vi "Set Enable Generic Event Flag.vi"(10 "Enable Generic Event Flag":bool, 11 "Template Server in":refnum<class "Template Server.lvclass">) -> (3 "Template Server out":refnum<class "Template Server.lvclass">)   [LabVIEW 2019, in "Template Server.lvlib" / "Template Server.lvclass"]
doc: "Enable the generic event if you would like to use a single event for capturing all messages. This would be useful if you are planning to implement your own dispatcher logic.\n\nKindly note that if generic event is enabled, individual events won't get generated."
uses:
  Template Server.lvclass
  Template Server.lvclass/Template Server.ctl
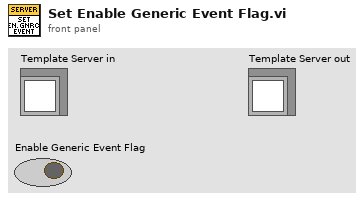
[diagram p1: front panel]
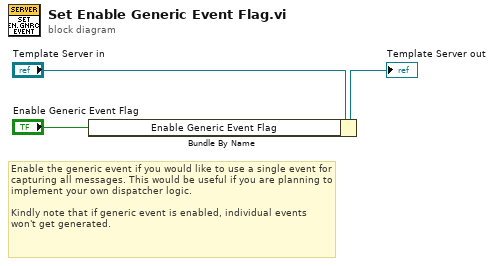
[diagram p0: block diagram]
diagram:
  # "Enable the generic event if you would like to use a single event for capturing all messages. This would be useful if you are planning to implement your own dispatcher logic.\n\nKindly note that if generic event is enabled, individual events won't get generated."
  n1 = Bundle By Name(cluster="Template Server in", "Enable Generic Event Flag"="Enable Generic Event Flag") -> (→"Template Server out":refnum<class "Template Server.lvclass">)
